vi "PH_PowerUnit_BaseClass.evt call Shot.vi"(0 "i ref in":refnum<vi>, 1 "PowerUnit":T1, 5 "error in (no error)":errorcluster) -> (14 "i ref out":refnum<vi>, 19 "error out":errorcluster)   [LabVIEW 2014, in "PH_PowerUnit_BaseClass.lvlib"]
doc: "This VI calls an event by a simple call."
uses:
  PH_PowerUnit_BaseClass.lvlib
  PH_PP_Common/PH_PP_Common.PUs.ctl
  CSCore/BaseProcess/BaseProcess.lvlib
  PH_PP_Common/PH_PP_Common.lvlib
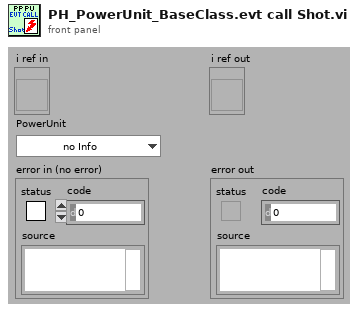
[diagram p1: front panel]
types:
  T1 = typedef "PH_PP_Common.lvlib/PH_PP_Common.PUs.ctl" = enum16{"no Info", "PA-19mm-1", "PA-19mm-2", "PA-45mm-PILC", "PA-45mm-MAIN", "MA-PU-1", "MA-PU-2", "MA-PU-3", "MA-PU-4", "MA-PU-5", "MA-PU-6", "MA-FR", "MA-PILC", "PA-45mm-DP"}
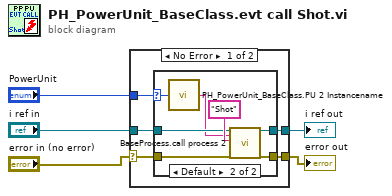
[diagram p0: block diagram]
diagram:
  n1 = case shown="No Error" "error in (no error)" {
    selector: "error in (no error)" -> [w6 w21]
    tunnel: [w10 w20] -> w5
    tunnel: [w9 w21] -> w4
    tunnel: "i ref in" -> [w8 w20]
    tunnel: "PowerUnit" -> [w7 _]
    frame No Error {
      n2 = case shown="Default" w7 {
        selector: w7 -> [_ w14]
        tunnel: [w12 w18] -> w10
        tunnel: [w11 w17] -> w9
        tunnel: w8 -> [w12 w16]
        tunnel: w6 -> [w11 w15]
        frame "no Info" {
        }
        frame Default {
          n3 = call "PH_PowerUnit_BaseClass.PU 2 Instancename.vi"("PU"=w14) -> ("Instance Name"=w13:string)
          n4 = call "BaseProcess.call process 2.vi"("i ref in"=w16, "Object"=w13, "Selector"="Shot", "error in (no error)"=w15) -> ("i ref out"=w18:refnum<vi>, "error out"=w17:errorcluster)  [unwired: 14 in]
        }
      }
    }
    frame Error {
    }
  }
  "i ref out" <- w5
  "error out" <- w4
